vi "Boolean Output Item Init.vi"(7 "Project In":refnum<class "Project.lvclass">, 8 "error in (no error)":errorcluster, 9 "Bool UI Elements":T1, 10 "Output":T2, 11 "VI in":refnum<vi>) -> (0 "error out":errorcluster)   [LabVIEW 2015, in "OutputUI.lvclass"]
uses:
  OutputUI.lvclass
  Step/STEP_OUTPUT.ctl
  Step/OUTPUT_DATA_TYPE.ctl
  OUTPUT_CHECK_TYPE.ctl
  Step/OUTPUT_VALUE_TYPE.ctl
  Project.lvclass
  Step.lvclass
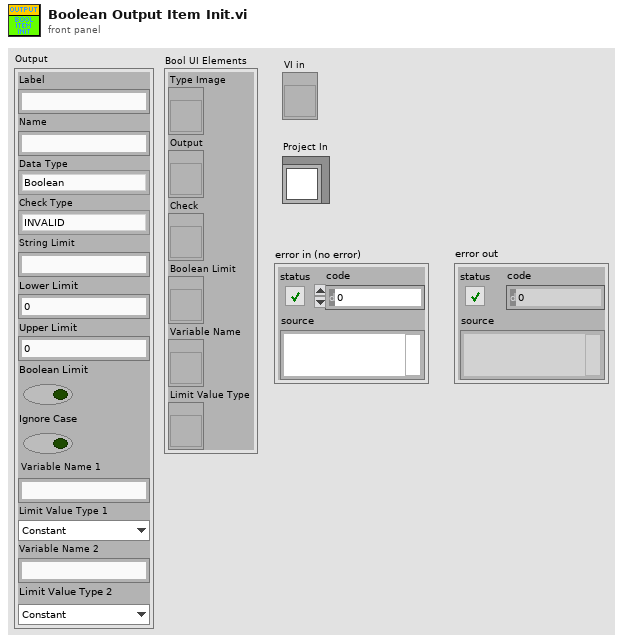
[diagram p1: front panel]
types:
  T1 = cluster{"Type Image":refnum<vi>, "Output":refnum<vi>, "Check":refnum<vi>, "Boolean Limit":refnum<vi>, "Variable Name":refnum<vi>, "Limit Value Type":refnum<vi>}
  T2 = typedef "Step.lvclass/STEP_OUTPUT.ctl" = cluster{"Label":string, "Name":string, "Data Type":T3, "Check Type":T4, "String Limit":string, "Lower Limit":dbl, "Upper Limit":dbl, "Boolean Limit":bool, "Ignore Case":bool, "Variable Name 1":string, "Limit Value Type 1":T5, "Variable Name 2":string, "Limit Value Type 2":T5}
  T3 = typedef "Step.lvclass/OUTPUT_DATA_TYPE.ctl" = enum16{"Boolean", "String", "Numeric", "Other"}
  T4 = typedef "Step.lvclass/OUTPUT_CHECK_TYPE.ctl" = enum16{"INVALID", "DO_NOT_CHECK", "RECORD", "VARIABLE", "EQUAL", "NOT_EQUAL", "STR_CONTAINS", "STR_START_WITH", "STR_END_WITH", "STR_REGEX_MATCH", "NUM_GT", "NUM_LT", "NUM_GE", "NUM_LE", "NUM_RANGE", "NUM_RANGE_BDY"}
  T5 = typedef "Step.lvclass/OUTPUT_VALUE_TYPE.ctl" = enum16{"Constant", "Variable"}
  T6 = cluster{"Type Image":refnum<vi>, "Output":refnum<vi>, "Check":refnum<vi>}
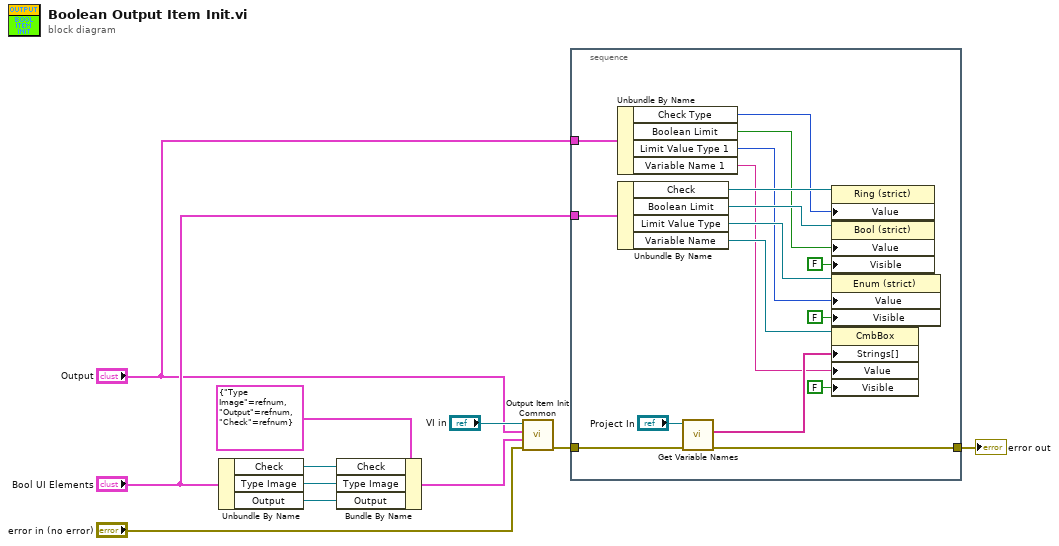
[diagram p0: block diagram]
diagram:
  n1 = Unbundle By Name("Bool UI Elements") -> ("Check"=w8:refnum<vi>, "Type Image"=w7:refnum<vi>, "Output"=w6:refnum<vi>)
  n2 = Bundle By Name(cluster=T6 {"Type Image"=refnum, "Output"=refnum, "Check"=refnum} ("UI Elements"), "Check"=w8, "Type Image"=w7, "Output"=w6) -> (w4:T6)
  n3 = call "Output Item Init Common.vi"("error in (no error)"="error in (no error)", "UI Elements"=w4, "Output"="Output", "VI in"="VI in") -> ("error out"=w1:errorcluster)  [unwired: 7 in]
  n4 = stacked-sequence {
    tunnel: "Output" -> [w28]
    tunnel: "Bool UI Elements" -> [w27]
    tunnel: w1 -> [w16]
    tunnel: [w15] -> w11
    frame #0 {
      n5 = Unbundle By Name(w28) -> ("Check Type"=w25:T4, "Boolean Limit"=w23:bool, "Limit Value Type 1"=w21:T5, "Variable Name 1"=w17:string)
      n6 = Unbundle By Name(w27) -> ("Check"=w26:refnum<vi>, "Boolean Limit"=w24:refnum<vi>, "Limit Value Type"=w22:refnum<vi>, "Variable Name"=w19:refnum<vi>)
      n7 = call "Get Variable Names.vi"("error in (no error)"=w16, "Project in"="Project In") -> ("error out"=w15:errorcluster, "Variable Names"=w18:string[])  [unwired: 7 in, 1 out]
      n8 = property class="Ring (strict)"(reference=w26, "Value"=w25) -> ()  [unwired: 1 in, 2 out]
      n9 = property class="Bool (strict)"(reference=w24, "Value"=w23, "Visible"=FALSE) -> ()  [unwired: 1 in, 2 out]
      n10 = property class="Enum (strict)"(reference=w22, "Value"=w21, "Visible"=FALSE) -> ()  [unwired: 1 in, 2 out]
      n11 = property class="CmbBox"(reference=w19, "Strings[]"=w18, "Value"=w17, "Visible"=FALSE) -> ()  [unwired: 1 in, 2 out]
    }
  }
  "error out" <- w11
